vi "Send event.vi"(0 "State":T2={"Prompt"="Click to add", "Listbox"=refnum, "Required"={"Strings"=[], "Bottom"=FALSE, "Italic"=FALSE, "FG"=0, "BG"=16777215, "Bold"=FALSE}, "Items"=[], "Req'd"=[], "Events"={"Items Changed"=refnum, "List Changed"=refnum}, "Max Rows"=-1, "Default name"=""}, 5 "Action":T1, 7 "Name":string, 9 "Start row":i32, 11 "End row":i32) -> ()   [LabVIEW 2020, in "KListboxEx.xctl"]
uses:
  KListboxEx.xctl
  State.ctl
  Required.ctl
  Events.ctl
  Event Action.ctl
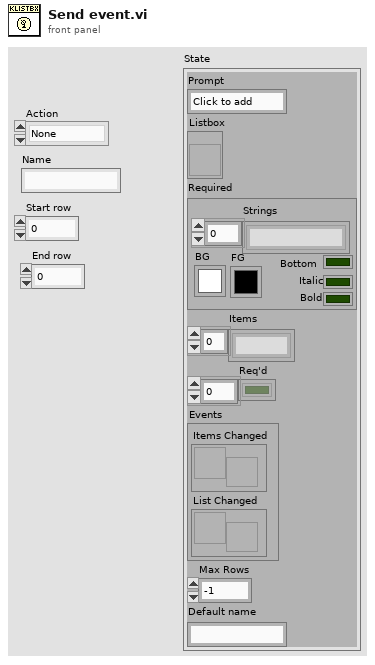
[diagram p1: front panel]
types:
  T1 = typedef "KListboxEx.xctl/Event Action.ctl" = enum16{"None", "Add", "Delete", "Move", "Edit", "Select"}
  T2 = typedef "KListboxEx.xctl/State.ctl" = cluster{"Prompt":string, "Listbox":refnum<vi>, "Required":T3, "Items":string[], "Req'd":bool[], "Events":T4, "Max Rows":i32, "Default name":string}
  T3 = typedef "KListboxEx.xctl/Required.ctl" = cluster{"Strings":string[], "Bottom":bool, "Italic":bool, "FG":u32, "BG":u32, "Bold":bool}
  T4 = typedef "KListboxEx.xctl/Events.ctl" = cluster{"Items Changed":refnum<user-event>, "List Changed":refnum<user-event>}
  T5 = cluster{"Action":T1, "Name":string, "Start row":i32, "End row":i32}
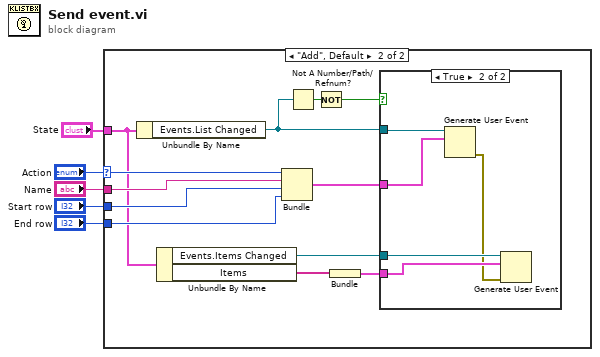
[diagram p0: block diagram]
diagram:
  n1 = case shown="\"Add\", Default" "Action" {
    selector: "Action" -> [_ w13]
    tunnel: "Name" -> [_ w12]
    tunnel: "Start row" -> [_ w11]
    tunnel: "End row" -> [_ w10]
    tunnel: "State" -> [_ w8]
    frame "None" {
    }
    frame "Add", Default {
      n2 = Unbundle By Name(w8) -> ("Events.List Changed"=w16:refnum<user-event>)
      n3 = Unbundle By Name(w8) -> ("Events.Items Changed"=w6:refnum<user-event>, "Items"=w7:string[])
      n4 = Bundle("Action"=w13, "Name"=w12, "Start row"=w11, "End row"=w10) -> (w9:T5)  [unwired: 1 in]
      n5 = Not A Number/Path/Refnum?(number/path/refnum=w16) -> (NaN/Path/Refnum?=w17:bool)
      n6 = Not(x=w17) -> (.not. x?=w14:bool)
      n7 = Bundle("Items"=w7) -> (w15:cluster{"Items":string[]})  [unwired: 1 in]
      n8 = case shown="True" w14 {
        tunnel: w16 -> [_ w18]
        tunnel: w15 -> [_ w20]
        tunnel: w9 -> [_ w22]
        tunnel: w6 -> [_ w21]
        frame False {
        }
        frame True {
          n9 = Generate User Event(user event=w18, event data cluster=w22) -> (error out=w19:errorcluster)  [unwired: 2 in, 1 out]
          n10 = Generate User Event(user event=w21, event data cluster=w20, error in=w19) -> ()  [unwired: 1 in, 2 out]
        }
      }
    }
  }
